vi "Set Max Heat Capacity.vi"(6 "parseError? T:Yes":bool=TRUE, 8 "error in (no error)":errorcluster, 10 "Maximum heating capacity(100%)":u8=100 max=100, 11 "VISA resource name":refnum<visa-resource-name>) -> (0 "error out":errorcluster, 3 "VISA resource name out":refnum<visa-resource-name>)   [LabVIEW 2015, in "JULABO DeviceDriver.lvlib"]
doc: "This VI adjusts the maximum allowed heating capacity in percent. 100 % corresponds to the technical specification of the equipment.\nAdustable range: <B>0 ... 100 %</B>\n\nValues outside the allowed range are coerced to fit the valid range and no error occurs."
uses:
  JULABO DeviceDriver.lvlib
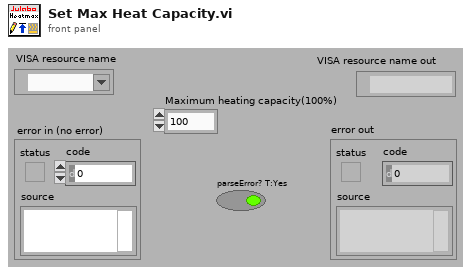
[diagram p1: front panel]
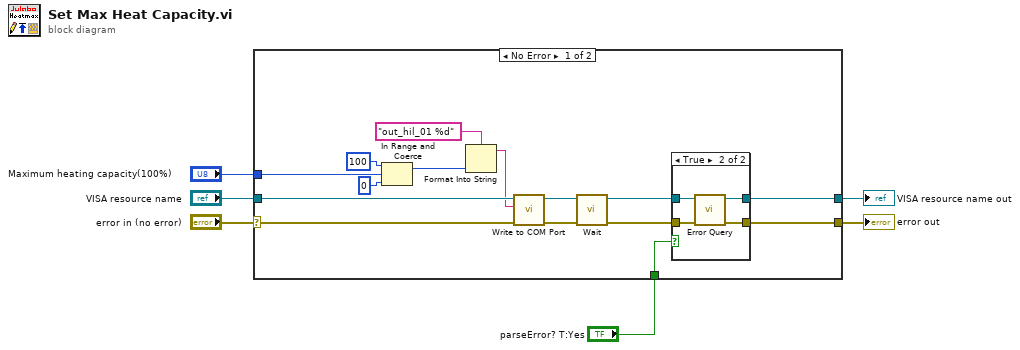
[diagram p0: block diagram]
diagram:
  n1 = case shown="No Error" "error in (no error)" {
    selector: "error in (no error)" -> [w20 w28]
    tunnel: "VISA resource name" -> [w21 w29]
    tunnel: [w19 w28] -> w5
    tunnel: [w18 w29] -> w4
    tunnel: "Maximum heating capacity(100%)" -> [w8 _]
    tunnel: "parseError? T:Yes" -> [w17 _]
    frame No Error {
      n2 = In Range and Coerce(upper limit=u8 100 ("oberer Grenzwert"), x=w8, lower limit=u8 0 ("unterer Grenzwert")) -> (coerced(x)=w7:u8)  [unwired: 1 out]
      n3 = Format Into String(format string="out_hil_01 %d", w7) -> (resulting string=w11:string)  [unwired: 2 in, 1 out]
      n4 = call "Write to COM Port.vi"("error in"=w20, "Command (input)"=w11, "VISA resource name in"=w21) -> ("error out"=w15:errorcluster, "VISA resource name out"=w16:refnum<visa-resource-name>)  [unwired: 7 in]
      n5 = call "Wait.vi"("error in"=w15, "VISA resource name in"=w16) -> ("error out"=w13:errorcluster, "VISA resource name out"=w14:refnum<visa-resource-name>)  [unwired: 4 in]
      n6 = case shown="True" w17 {
        tunnel: w14 -> [w23 w27]
        tunnel: w13 -> [w22 w26]
        tunnel: [w23 w25] -> w18
        tunnel: [w22 w24] -> w19
        frame False {
        }
        frame True {
          n7 = call "Error Query.vi"("error in (no error)"=w26, "VISA resource name"=w27) -> ("error out"=w24:errorcluster, "VISA resource name out"=w25:refnum<visa-resource-name>)  [unwired: 6 in, 2 out]
        }
      }
    }
    frame Error {
    }
  }
  "error out" <- w5
  "VISA resource name out" <- w4
